vi "OrganizeSubroutines.vi"(1 "URAPI Script":T1={"Script"="", "Whiles"=[], "Ifs"=[], "Supress Err"=TRUE, "Errors"=""}) -> (0 "URAPI Script":T1={"Script"="", "Whiles"=[], "Ifs"=[], "Supress Err"=TRUE, "Errors"=""})   [LabVIEW 2012]
uses:
  <userlib>/BotSpeak/VIs/Direct/URAPI_Control.ctl
panel:
  out "subs":string[](array[string])
  out "Subs":string[](array[string])
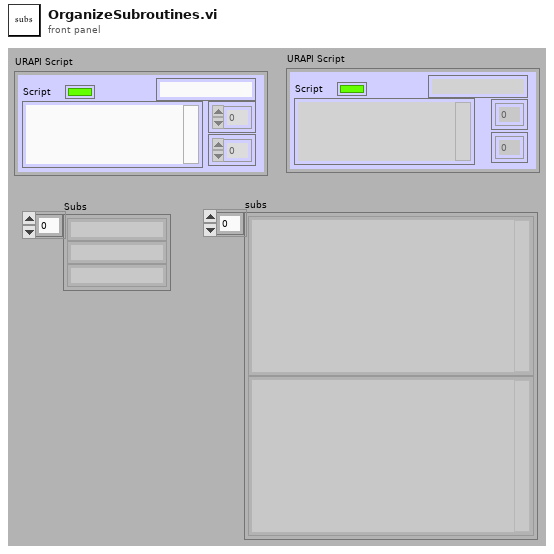
[diagram p1: front panel]
types:
  T1 = typedef "URAPI_Control.ctl" = cluster{"Script":string, "Whiles":u8[], "Ifs":u8[], "Supress Err":bool, "Errors":string}
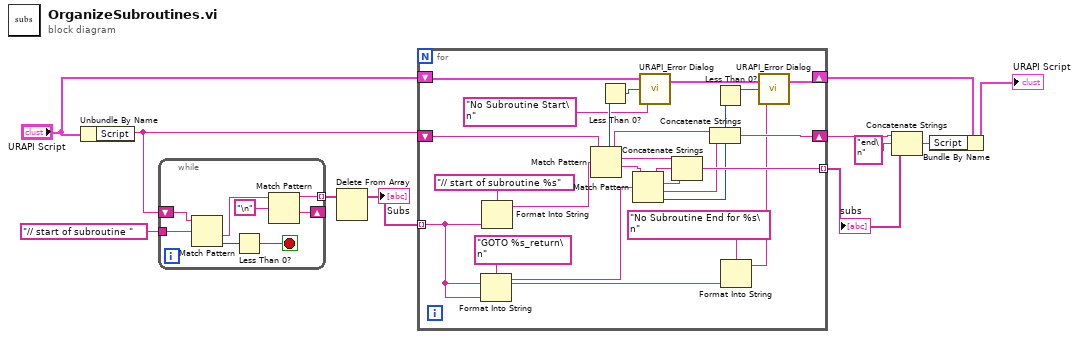
[diagram p0: block diagram]
diagram:
  n1 = Unbundle By Name("URAPI Script") -> ("Script"=w5:string)
  n2 = while {
    shift-right: [w14] -> _
    shift-left: w5 -> [w19]
    tunnel: "// start of subroutine " ("regular expression") -> [w18]
    tunnel: [w15] -> w10 mode=indexing
    stop <- w12 stop-if-true
    n3 = Match Pattern(string=w19, regular expression=w18) -> (after substring=w17:string, offset past match=w13:i32)  [unwired: 1 in, 2 out]
    n4 = Less Than 0?(x=w13) -> (x < 0?=w12:bool)
    n5 = Match Pattern(string=w17, regular expression="\n") -> (before substring=w15:string, after substring=w14:string)  [unwired: 1 in, 2 out]
  }
  n6 = Delete From Array(array=w10) -> (array with subset deleted=w9:string[])  [unwired: 2 in, 1 out]
  "Subs" <- w9
  n7 = for {
    shift-right: [w31] -> w8
    shift-left: w5 -> [w42]
    tunnel: w9 -> [w22] mode=indexing
    tunnel: [w34] -> w6 mode=indexing
    shift-right: [w25] -> w3
    shift-left: "URAPI Script" -> [w27]
    n8 = Format Into String(format string="GOTO %s_return\n" ("regular expression"), w22) -> (resulting string=w39:string)  [unwired: 2 in, 1 out]
    n9 = Format Into String(format string="// start of subroutine %s" ("regular expression"), w22) -> (resulting string=w41:string)  [unwired: 2 in, 1 out]
    n10 = Match Pattern(string=w42, regular expression=w41) -> (before substring=w33:string, match substring=w38:string, after substring=w37:string, offset past match=w30:i32)  [unwired: 1 in]
    n11 = Less Than 0?(x=w30) -> (x < 0?=w28:bool)
    n12 = Match Pattern(string=w37, regular expression=w39) -> (before substring=w36:string, match substring=w35:string, after substring=w32:string, offset past match=w29:i32)  [unwired: 1 in]
    n13 = call <userlib>:"URAPI_Error Dialog.vi"("Error String"="No Subroutine Start\n", "Error?"=w28, "URAPI Script in"=w27) -> ("URAPI Script out"=w24:T1)  [unwired: 1 in]
    n14 = Concatenate Strings(w38, w36, w35) -> (w34:string)
    n15 = Concatenate Strings(w33, w32) -> (w31:string)
    n16 = Less Than 0?(x=w29) -> (x < 0?=w23:bool)
    n17 = Format Into String(format string="No Subroutine End for %s\n" ("Error String"), w22) -> (resulting string=w20:string)  [unwired: 2 in, 1 out]
    n18 = call <userlib>:"URAPI_Error Dialog.vi"("Error String"=w20, "Error?"=w23, "URAPI Script in"=w24) -> ("URAPI Script out"=w25:T1)  [unwired: 1 in]
  }
  "subs" <- w6
  n19 = Concatenate Strings(w8, "end\n" ("string"), w6) -> (w1:string)
  n20 = Bundle By Name(cluster=w3, "Script"=w1) -> (→"URAPI Script":T1)
